vi "LSMcontroller_v61_updatedROIselection.vi"() -> ()   [LabVIEW 2015] (continued)
                  frame False {
                  }
                  frame True {
                    n4769 = local read "Meastab"() -> (w1613:enum32{"X-Y Image", "Linescan", "Timetrace"})
                    n4770 = call "waveformparamsv2.vi"("command"="get") -> ("Params out"=w1619:T15)  [unwired: 4 in, 2 out]
                    n4771 = Unbundle By Name(w1619) -> ("AO parameters"=w1618:T16)
                    n4772 = case shown="\"Timetrace\"" w1613 {
                      tunnel: [w1633 w1634] -> w1612
                      frame "X-Y Image", Default {
                        n4773 = local read "Sampling rate"() -> (w1633:dbl)
                      }
                      frame "Timetrace" {
                        n4774 = local read "srateAODOtt"() -> (w1634:dbl)
                      }
                    }
                    n4775 = Index Array(array=w1618, index=w1616) -> (element=w1617:T17)
                    n4776 = call "waveformsAObuffer.vi"("command"="get") -> ("AO wf out"=w1623:waveform(dbl)[])  [unwired: 1 in]
                    n4777 = call "matlabAOwffromparam.vi"("Cluster"=w1617) -> ("Waveform"=w1621:waveform(dbl))  [unwired: 1 out]
                    n4778 = property on="refwf" class="Ring (strict)"() -> ("RingText.Text"=w1624:string)  [unwired: 2 in, 2 out]
                    n4779 = Replace Array Subset(array=w1623, new element=w1621, index=w1616) -> (w1622:waveform(dbl)[])
                    n4780 = call "waveformsDObuffer.vi"("command"="get") -> ("DO wf out"=w1629:digitalwaveform[])  [unwired: 1 in]
                    n4781 = call "correctwaveformsizetemp.vi"("new sampling frequency (Hz)"=w1612, "start"=FALSE, "reference waveforms to"=w1624, "Analog waveforms in"=w1622, "stop"=FALSE, "Digital waveforms in"=w1629) -> ("analog wf out"=w1627:waveform(dbl)[], "Digital wf out"=w1625:digitalwaveform[], "measpoints"=w1614:i32)
                    n4782 = local read "wavdet"() -> (w1615:bool)
                    n4783 = local write "Analog Lines Plot"(w1627) -> ()
                    n4784 = call "GetNumCamFramesv2.vi"("Digital Waveform Graph"=w1625) -> ("Numeric"=w1626:i32)  [unwired: 10 in]
                    n4785 = local write "Digital Lines Plot"(w1625) -> ()
                    n4786 = call "waveformsAObuffer.vi"("AO wf in"=w1627, "command"="set") -> ()  [unwired: 1 out]
                    n4787 = call "waveformsDObuffer.vi"("DO wf in"=w1625, "command"="set") -> ()  [unwired: 1 out]
                    n4788 = local write "Total Camera Frames"(w1626) -> ()
                    n4789 = case shown="True" w1615 {
                      tunnel: w1614 -> [_ w1635]
                      frame False {
                      }
                      frame True {
                        n4790 = local write "# of frames"(w1635) -> ()
                      }
                    }
                  }
                }
              }
              frame #4 {
                n4791 = local read "finite samples"() -> (w1636:bool)
                n4792 = local read "continuous"() -> (w1637:bool)
                n4793 = local read "wavdet"() -> (w1638:bool)
                n4794 = call "2pparameters.vi"("command"="get") -> ("params out"=w1641:T11)  [unwired: 1 in]
                n4795 = Bundle By Name(cluster=w1641, "finite"=w1636, "cont"=w1637, "wavdet"=w1638) -> (w1639:T11)
                n4796 = call "2pparameters.vi"("Params in"=w1639, "command"="set") -> ()  [unwired: 1 out]
              }
            }
          }
          event "Load Matlab Waveform DO": Value Change {
            n4797 = event-data() -> ()  [unwired: 1 in, 6 out]
            n4798 = stacked-sequence {
              seq-local: [_ _ w1749 _ _] -> [_ _ _ w1764 _]
              seq-local: [_ _ w1748 _ _] -> [_ _ _ w1763 _]
              frame #0 {
                n4799 = local read "Measurement"() -> (w1643:T4)
                n4800 = case shown="\"X-Y-t movie\", Default" w1643 {
                  frame "X-Y-t movie", Default {
                    n4801 = local read "avpp"() -> (w1664:i32)
                    n4802 = local read "Angle ref"() -> (w1663:dbl)
                    n4803 = local read "ROI Type"() -> (w1662:u16)
                    n4804 = local read "xpixels ref"() -> (w1659:i32)
                    n4805 = local read "Vx-min ref"() -> (w1658:dbl)
                    n4806 = local read "Vx-max ref"() -> (w1657:dbl)
                    n4807 = local read "ypixels ref"() -> (w1655:i32)
                    n4808 = local read "Vy-min ref"() -> (w1656:dbl)
                    n4809 = local read "Vy-max ref"() -> (w1652:dbl)
                    n4810 = local read "Sampling rate"() -> (w1646:dbl)
                    n4811 = local read "finite samples"() -> (w1647:bool)
                    n4812 = local read "continuous"() -> (w1650:bool)
                    n4813 = local read "wavdet"() -> (w1651:bool)
                    n4814 = local read "# of frames"() -> (w1649:i32)
                    n4815 = local read "maxbufferAI"() -> (w1648:i32)
                    n4816 = local read "Override AI buffer"() -> (w1644:bool)
                    n4817 = call "2pparameters.vi"("command"="get") -> ("params out"=w1661:T11)  [unwired: 1 in]
                    n4818 = Bundle By Name(cluster=w1661, "type"="X-Y-t movie", "avpp"=w1664, "Angle Img"=w1663, "Xpixels Img"=w1659, "Vx-min Img"=w1658, "VX-max Img"=w1657, "Ypixels Img"=w1655, "Vy-min Img"=w1656, "Vy-max Img"=w1652, "srate"=w1646, "srate Img"=w1646, "finite"=w1647, "cont"=w1650, "wavdet"=w1651, "measpoints"=w1649, "maxbufferAI"=w1648, "Drawing Mode"=w1662, "Vz-reset"=0.0, "AIoverride"=w1644) -> (w1653:T11)
                    n4819 = call "2pparameters.vi"("Params in"=w1653, "command"="set") -> ()  [unwired: 1 out]
                  }
                  frame "X-Y-Z stack" {
                    n4820 = call "2pparameters.vi"("command"="get") -> ("params out"=w1668:T11)  [unwired: 1 in]
                    n4821 = Bundle By Name(cluster=w1668, "type"="X-Y-Z stack") -> (w1666:T11)
                    n4822 = call "2pparameters.vi"("Params in"=w1666, "command"="set") -> ()  [unwired: 1 out]
                  }
                  frame "Lifetime (scan)" {
                    n4823 = call "2pparameters.vi"("command"="get") -> ("params out"=w1673:T11)  [unwired: 1 in]
                    n4824 = Bundle By Name(cluster=w1673, "type"="Lifetime (scan)") -> (w1671:T11)
                    n4825 = call "2pparameters.vi"("Params in"=w1671, "command"="set") -> ()  [unwired: 1 out]
                  }
                  frame "Lifetime (contour)" {
                    n4826 = local read "Vy-min draw"() -> (w1683:dbl)
                    n4827 = local read "Vy-max draw"() -> (w1682:dbl)
                    n4828 = local read "Vx-min draw"() -> (w1685:dbl)
                    n4829 = local read "Vx-max draw"() -> (w1684:dbl)
                    n4830 = local read "xpixels ref"() -> (w1681:i32)
                    n4831 = local read "ypixels ref"() -> (w1680:i32)
                    n4832 = local read "ROI Type"() -> (w1679:u16)
                    n4833 = local read "srateAODOtt"() -> (w1690:dbl)
                    n4834 = local read "# of frames"() -> (w1695:i32)
                    n4835 = local read "refreshtime"() -> (w1687:dbl)
                    n4836 = local read "Pel"() -> (w1678:dbl)
                    n4837 = local read "bin"() -> (w1693:dbl)
                    n4838 = local read "Override AI buffer"() -> (w1676:bool)
                    n4839 = local read "finite samples"() -> (w1702:bool)
                    n4840 = local read "srateAODOtt"() -> (w1689:dbl)
                    n4841 = local read "srateAODOtt"() -> (w1696:dbl)
                    n4842 = local read "continuous"() -> (w1701:bool)
                    n4843 = local read "Angle ref"() -> (w1686:dbl)
                    n4844 = local read "wavdet"() -> (w1703:bool)
                    n4845 = local read "Vx-ref"() -> (w1698:dbl)
                    n4846 = local read "Vy-ref"() -> (w1700:dbl)
                    n4847 = local read "avpp"() -> (w1699:i32)
                    n4848 = call "tt_timeandsamples.vi"("bin"=w1693, "refreshtime"=w1687, "srateAODOtt"=w1690, "tot#ofsamples"=w1695) -> ("refreshrate"=w1691:dbl, "refreshbuffer"=w1692:i32, "timetracecycles"=w1697:i32)  [unwired: 5 in]
                    n4849 = local read "bin"() -> (w1694:dbl)
                    n4850 = call "2pparameters.vi"("command"="get") -> ("params out"=w1706:T11)  [unwired: 1 in]
                    n4851 = Bundle By Name(cluster=w1706, "Drawing Mode"=w1679, "measpoints"=w1695, "tt_cycles"=w1697, "refreshbuffer"=w1692, "refreshrate"=w1691, "Vx-ref"=w1698, "Vy-ref"=w1700, "srate"=w1689, "finite"=w1702, "cont"=w1701, "wavdet"=w1703, "avpp"=w1699, "srateAODO"=w1696, "bufferAI"=w1692, "bin"=w1694, "Angle Img"=w1686, "Vxminref"=w1685, "Vxmaxref"=w1684, "Vyminref"=w1683, "Vymaxref"=w1682, "Xpixels Img"=w1681, "Ypixels Img"=w1680, "Pel"=w1678, "Vz-reset"=0.0, "AIoverride"=w1676, "type"="Lifetime (contour)") -> (w1704:T11)
                    n4852 = Reciprocal(x=w1691) -> (1/x=w1688:dbl)
                    n4853 = local write "refreshtime"(w1688) -> ()
                    n4854 = call "2pparameters.vi"("Params in"=w1704, "command"="set") -> ()  [unwired: 1 out]
                  }
                  frame "X-Y-Z-t movie" {
                  }
                  frame "linescan" {
                  }
                  frame "Timetrace" {
                    n4855 = local read "Vy-min draw"() -> (w1716:dbl)
                    n4856 = local read "Vy-max draw"() -> (w1715:dbl)
                    n4857 = local read "Vx-min draw"() -> (w1718:dbl)
                    n4858 = local read "Vx-max draw"() -> (w1717:dbl)
                    n4859 = local read "xpixels ref"() -> (w1714:i32)
                    n4860 = local read "ypixels ref"() -> (w1713:i32)
                    n4861 = local read "ROI Type"() -> (w1712:u16)
                    n4862 = local read "srateAODOtt"() -> (w1723:dbl)
                    n4863 = local read "# of frames"() -> (w1728:i32)
                    n4864 = local read "refreshtime"() -> (w1720:dbl)
                    n4865 = local read "Pel"() -> (w1711:dbl)
                    n4866 = local read "bin"() -> (w1726:dbl)
                    n4867 = local read "Override AI buffer"() -> (w1709:bool)
                    n4868 = local read "finite samples"() -> (w1735:bool)
                    n4869 = local read "srateAODOtt"() -> (w1722:dbl)
                    n4870 = local read "srateAODOtt"() -> (w1729:dbl)
                    n4871 = local read "continuous"() -> (w1734:bool)
                    n4872 = local read "Angle ref"() -> (w1719:dbl)
                    n4873 = local read "wavdet"() -> (w1736:bool)
                    n4874 = local read "Vx-ref"() -> (w1731:dbl)
                    n4875 = local read "Vy-ref"() -> (w1733:dbl)
                    n4876 = local read "avpp"() -> (w1732:i32)
                    n4877 = call "tt_timeandsamples.vi"("bin"=w1726, "refreshtime"=w1720, "srateAODOtt"=w1723, "tot#ofsamples"=w1728) -> ("refreshrate"=w1724:dbl, "refreshbuffer"=w1725:i32, "timetracecycles"=w1730:i32)  [unwired: 5 in]
                    n4878 = local read "bin"() -> (w1727:dbl)
                    n4879 = call "2pparameters.vi"("command"="get") -> ("params out"=w1739:T11)  [unwired: 1 in]
                    n4880 = Bundle By Name(cluster=w1739, "Drawing Mode"=w1712, "measpoints"=w1728, "tt_cycles"=w1730, "refreshbuffer"=w1725, "refreshrate"=w1724, "Vx-ref"=w1731, "Vy-ref"=w1733, "srate"=w1722, "finite"=w1735, "cont"=w1734, "wavdet"=w1736, "avpp"=w1732, "srateAODO"=w1729, "bufferAI"=w1725, "bin"=w1727, "Angle Img"=w1719, "Vxminref"=w1718, "Vxmaxref"=w1717, "Vyminref"=w1716, "Vymaxref"=w1715, "Xpixels Img"=w1714, "Ypixels Img"=w1713, "Pel"=w1711, "Vz-reset"=0.0, "AIoverride"=w1709, "type"="Timetrace") -> (w1737:T11)
                    n4881 = Reciprocal(x=w1724) -> (1/x=w1721:dbl)
                    n4882 = local write "refreshtime"(w1721) -> ()
                    n4883 = call "2pparameters.vi"("Params in"=w1737, "command"="set") -> ()  [unwired: 1 out]
                  }
                  frame "Lifetime (point)" {
                  }
                }
              }
              frame #1 {
                w1742 = FALSE ("wavdet")
                n4884 = call "2pparameters.vi"("command"="get") -> ("params out"=w1746:T11)  [unwired: 1 in]
                n4885 = Bundle By Name(cluster=w1746, "finite"=w1742, "cont"=w1742, "wavdet"=TRUE) -> (w1743:T11)
                n4886 = call "2pparameters.vi"("Params in"=w1743, "command"="set") -> ()  [unwired: 1 out]
              }
              frame #2 {
                n4887 = local read "DO channels"() -> (w1751:u16)
                n4888 = call "2pparameters.vi"("command"="get") -> ("params out"=w1753:T11)  [unwired: 1 in]
                n4889 = Unbundle By Name(w1753) -> ("aDO"=w1752:u32[])
                n4890 = Search 1D Array(1D array=w1752, element=w1751) -> (index of element=w1749:i32)  [unwired: 1 in]
                n4891 = Greater?(x=w1749, y=-1) -> (0:w1748:bool)
                n4892 = case shown="True" w1748 {
                  tunnel: w1749 -> [_ w1760]
                  frame False {
                  }
                  frame True {
                    n4893 = local read "Meastab"() -> (w1756:enum32{"X-Y Image", "Linescan", "Timetrace"})
                    n4894 = local read "Matlab waveform path DO"() -> (w1758:path)
                    n4895 = local read "Matlab padding value DO"() -> (w1759:dbl)
                    n4896 = case shown="\"Timetrace\"" w1756 {
                      tunnel: [w1761 w1762] -> w1755
                      frame "X-Y Image", Default {
                        n4897 = local read "Sampling rate"() -> (w1761:dbl)
                      }
                      frame "Timetrace" {
                        n4898 = local read "srateAODOtt"() -> (w1762:dbl)
                      }
                    }
                    n4899 = call "matlabwfexistsdialogue.vi"("Matlab waveform path"=w1758) -> ("mtalab waveform path out"=w1757:path)
                    n4900 = call "replace DO matlab param.vi"("Sampling frequency (Hz)"=w1755, "matlab wave number"=w1757, "index of DO wave"=w1760, "padding value"=w1759) -> ()  [unwired: 7 in]
                  }
                }
              }
              frame #3 {
                n4901 = case shown="True" w1763 {
                  tunnel: w1764 -> [_ w1773]
                  frame False {
                  }
                  frame True {
                    n4902 = local read "Meastab"() -> (w1768:enum32{"X-Y Image", "Linescan", "Timetrace"})
                    n4903 = call "waveformparamsv2.vi"("command"="get") -> ("Params out"=w1786:T15)  [unwired: 4 in, 2 out]
                    n4904 = Unbundle By Name(w1786) -> ("DO parameters"=w1785:T18)
                    n4905 = case shown="\"Timetrace\"" w1768 {
                      tunnel: [w1788 w1789] -> w1767
                      frame "X-Y Image", Default {
                        n4906 = local read "Sampling rate"() -> (w1788:dbl)
                      }
                      frame "Timetrace" {
                        n4907 = local read "srateAODOtt"() -> (w1789:dbl)
                      }
                    }
                    n4908 = Index Array(array=w1785, index=w1773) -> (element=w1772:T19)
                    n4909 = call "waveformsDObuffer.vi"("command"="get") -> ("DO wf out"=w1783:digitalwaveform[])  [unwired: 1 in]
                    n4910 = property on="refwf" class="Ring (strict)"() -> ("RingText.Text"=w1775:string)  [unwired: 2 in, 2 out]
                    n4911 = call "matlabDOwffromparam.vi"("waveform params"=w1772) -> ("digital waveform"=w1771:digitalwaveform)
                    n4912 = Replace Array Subset(array=w1783, new element=w1771, index=w1773) -> (w1774:digitalwaveform[])
                    n4913 = call "waveformsAObuffer.vi"("command"="get") -> ("AO wf out"=w1782:waveform(dbl)[])  [unwired: 1 in]
                    n4914 = local read "wavdet"() -> (w1770:bool)
                    n4915 = call "correctwaveformsizetemp.vi"("new sampling frequency (Hz)"=w1767, "start"=FALSE, "reference waveforms to"=w1775, "Analog waveforms in"=w1782, "stop"=FALSE, "Digital waveforms in"=w1774) -> ("analog wf out"=w1778:waveform(dbl)[], "Digital wf out"=w1776:digitalwaveform[], "measpoints"=w1769:i32)
                    n4916 = local write "Analog Lines Plot"(w1778) -> ()
                    n4917 = call "GetNumCamFramesv2.vi"("Digital Waveform Graph"=w1776) -> ("Numeric"=w1777:i32)  [unwired: 10 in]
                    n4918 = local write "Digital Lines Plot"(w1776) -> ()
                    n4919 = case shown="True" w1770 {
                      tunnel: w1769 -> [_ w1790]
                      frame False {
                      }
                      frame True {
                        n4920 = local write "# of frames"(w1790) -> ()
                      }
                    }
                    n4921 = call "waveformsAObuffer.vi"("AO wf in"=w1778, "command"="set") -> ()  [unwired: 1 out]
                    n4922 = call "waveformsDObuffer.vi"("DO wf in"=w1776, "command"="set") -> ()  [unwired: 1 out]
                    n4923 = local write "Total Camera Frames"(w1777) -> ()
                  }
                }
              }
              frame #4 {
                n4924 = local read "finite samples"() -> (w1791:bool)
                n4925 = local read "continuous"() -> (w1792:bool)
                n4926 = local read "wavdet"() -> (w1793:bool)
                n4927 = call "2pparameters.vi"("command"="get") -> ("params out"=w1796:T11)  [unwired: 1 in]
                n4928 = Bundle By Name(cluster=w1796, "finite"=w1791, "cont"=w1792, "wavdet"=w1793) -> (w1794:T11)
                n4929 = call "2pparameters.vi"("Params in"=w1794, "command"="set") -> ()  [unwired: 1 out]
              }
            }
          }
          event "Add settings": Value Change {
            n4930 = event-data() -> ()  [unwired: 1 in, 6 out]
            n4931 = call "wfsettings.vi"("command"="get") -> ("wfsettings out"=w1800:T29)  [unwired: 2 in, 1 out]
            n4932 = in-place {
              n4933 = in-place-cluster #53(w1800) -> ("settings names"=w1805:string[], "settings locations"=w1807:path[])
              n4934 = local read "Setting location"() -> (w1803:path)
              n4935 = local read "Nickname"() -> (w1802:string)
              n4936 = Build Array (concatenate)(w1805, w1802) -> (w1804:string[])
              n4937 = property on="Loaded settings" class="Ring (strict)"("Strings []"=w1804) -> ()  [unwired: 2 in, 2 out]
              n4938 = Build Array (concatenate)(w1807, w1803) -> (w1806:path[])
              n4939 = in-place-cluster #53("settings names"=w1804, "settings locations"=w1806) -> (w1798:T29)
            }
            n4940 = call "wfsettings.vi"("wfsettings in"=w1798, "command"="set") -> ()  [unwired: 1 in, 2 out]
          }
          event "Rem setting": Value Change {
            n4941 = event-data() -> ()  [unwired: 1 in, 6 out]
            n4942 = call "wfsettings.vi"("command"="get") -> ("wfsettings out"=w1810:T29)  [unwired: 2 in, 1 out]
            n4943 = in-place {
              n4944 = in-place-cluster #54(w1810) -> ("settings names"=w1815:string[], "settings locations"=w1813:path[])
              n4945 = property on="Loaded settings" class="Ring (strict)"() -> ("RingText.Text"=w1816:string)  [unwired: 2 in, 2 out]
              n4946 = Search 1D Array(1D array=w1815, element=w1816) -> (index of element=w1817:i32)  [unwired: 1 in]
              n4947 = Delete From Array(array=w1815, index=w1817) -> (array with subset deleted=w1814:string[])  [unwired: 1 in, 1 out]
              n4948 = Delete From Array(array=w1813, index=w1817) -> (array with subset deleted=w1812:path[])  [unwired: 1 in, 1 out]
              n4949 = property on="Loaded settings" class="Ring (strict)"("Strings []"=w1814) -> ()  [unwired: 2 in, 2 out]
              n4950 = in-place-cluster #54("settings names"=w1814, "settings locations"=w1812) -> (w1808:T29)
            }
            n4951 = call "wfsettings.vi"("wfsettings in"=w1808, "command"="set") -> ()  [unwired: 1 in, 2 out]
          }
          event "Update settings": Value Change {
            n4952 = event-data() -> ()  [unwired: 1 in, 6 out]
            n4953 = stacked-sequence {
              frame #0 {
                n4954 = local read "Measurement"() -> (w1818:T4)
                n4955 = case shown="\"Timetrace\"" w1818 {
                  frame "X-Y-t movie", Default {
                    n4956 = local read "avpp"() -> (w1839:i32)
                    n4957 = local read "Angle ref"() -> (w1838:dbl)
                    n4958 = local read "ROI Type"() -> (w1837:u16)
                    n4959 = local read "xpixels ref"() -> (w1834:i32)
                    n4960 = local read "Vx-min ref"() -> (w1833:dbl)
                    n4961 = local read "Vx-max ref"() -> (w1832:dbl)
                    n4962 = local read "ypixels ref"() -> (w1830:i32)
                    n4963 = local read "Vy-min ref"() -> (w1831:dbl)
                    n4964 = local read "Vy-max ref"() -> (w1827:dbl)
                    n4965 = local read "Sampling rate"() -> (w1821:dbl)
                    n4966 = local read "finite samples"() -> (w1822:bool)
                    n4967 = local read "continuous"() -> (w1825:bool)
                    n4968 = local read "wavdet"() -> (w1826:bool)
                    n4969 = local read "# of frames"() -> (w1824:i32)
                    n4970 = local read "maxbufferAI"() -> (w1823:i32)
                    n4971 = local read "Override AI buffer"() -> (w1819:bool)
                    n4972 = call "2pparameters.vi"("command"="get") -> ("params out"=w1836:T11)  [unwired: 1 in]
                    n4973 = Bundle By Name(cluster=w1836, "type"="X-Y-t movie", "avpp"=w1839, "Angle Img"=w1838, "Xpixels Img"=w1834, "Vx-min Img"=w1833, "VX-max Img"=w1832, "Ypixels Img"=w1830, "Vy-min Img"=w1831, "Vy-max Img"=w1827, "srate"=w1821, "srate Img"=w1821, "finite"=w1822, "cont"=w1825, "wavdet"=w1826, "measpoints"=w1824, "maxbufferAI"=w1823, "Drawing Mode"=w1837, "Vz-reset"=0.0, "AIoverride"=w1819) -> (w1828:T11)
                    n4974 = call "2pparameters.vi"("Params in"=w1828, "command"="set") -> ()  [unwired: 1 out]
                  }
                  frame "X-Y-Z stack" {
                    n4975 = call "2pparameters.vi"("command"="get") -> ("params out"=w1843:T11)  [unwired: 1 in]
                    n4976 = Bundle By Name(cluster=w1843, "type"="X-Y-Z stack") -> (w1841:T11)
                    n4977 = call "2pparameters.vi"("Params in"=w1841, "command"="set") -> ()  [unwired: 1 out]
                  }
                  frame "Lifetime (scan)" {
                    n4978 = call "2pparameters.vi"("command"="get") -> ("params out"=w1848:T11)  [unwired: 1 in]
                    n4979 = Bundle By Name(cluster=w1848, "type"="Lifetime (scan)") -> (w1846:T11)
                    n4980 = call "2pparameters.vi"("Params in"=w1846, "command"="set") -> ()  [unwired: 1 out]
                  }
                  frame "Lifetime (contour)" {
                    n4981 = local read "Vy-min draw"() -> (w1858:dbl)
                    n4982 = local read "Vy-max draw"() -> (w1857:dbl)
                    n4983 = local read "Vx-min draw"() -> (w1860:dbl)
                    n4984 = local read "Vx-max draw"() -> (w1859:dbl)
                    n4985 = local read "xpixels ref"() -> (w1856:i32)
                    n4986 = local read "ypixels ref"() -> (w1855:i32)
                    n4987 = local read "ROI Type"() -> (w1854:u16)
                    n4988 = local read "srateAODOtt"() -> (w1865:dbl)
                    n4989 = local read "# of frames"() -> (w1870:i32)
                    n4990 = local read "refreshtime"() -> (w1862:dbl)
                    n4991 = local read "Pel"() -> (w1853:dbl)
                    n4992 = local read "bin"() -> (w1868:dbl)
                    n4993 = local read "Override AI buffer"() -> (w1851:bool)
                    n4994 = local read "finite samples"() -> (w1877:bool)
                    n4995 = local read "srateAODOtt"() -> (w1864:dbl)
                    n4996 = local read "srateAODOtt"() -> (w1871:dbl)
                    n4997 = local read "continuous"() -> (w1876:bool)
                    n4998 = local read "Angle ref"() -> (w1861:dbl)
                    n4999 = local read "wavdet"() -> (w1878:bool)
                    n5000 = local read "Vx-ref"() -> (w1873:dbl)
                    n5001 = local read "Vy-ref"() -> (w1875:dbl)
                    n5002 = local read "avpp"() -> (w1874:i32)
                    n5003 = call "tt_timeandsamples.vi"("bin"=w1868, "refreshtime"=w1862, "srateAODOtt"=w1865, "tot#ofsamples"=w1870) -> ("refreshrate"=w1866:dbl, "refreshbuffer"=w1867:i32, "timetracecycles"=w1872:i32)  [unwired: 5 in]
                    n5004 = local read "bin"() -> (w1869:dbl)
                    n5005 = call "2pparameters.vi"("command"="get") -> ("params out"=w1881:T11)  [unwired: 1 in]
                    n5006 = Bundle By Name(cluster=w1881, "Drawing Mode"=w1854, "measpoints"=w1870, "tt_cycles"=w1872, "refreshbuffer"=w1867, "refreshrate"=w1866, "Vx-ref"=w1873, "Vy-ref"=w1875, "srate"=w1864, "finite"=w1877, "cont"=w1876, "wavdet"=w1878, "avpp"=w1874, "srateAODO"=w1871, "bufferAI"=w1867, "bin"=w1869, "Angle Img"=w1861, "Vxminref"=w1860, "Vxmaxref"=w1859, "Vyminref"=w1858, "Vymaxref"=w1857, "Xpixels Img"=w1856, "Ypixels Img"=w1855, "Pel"=w1853, "Vz-reset"=0.0, "AIoverride"=w1851, "type"="Lifetime (contour)") -> (w1879:T11)
                    n5007 = Reciprocal(x=w1866) -> (1/x=w1863:dbl)
                    n5008 = local write "refreshtime"(w1863) -> ()
                    n5009 = call "2pparameters.vi"("Params in"=w1879, "command"="set") -> ()  [unwired: 1 out]
                  }
                  frame "X-Y-Z-t movie" {
                  }
                  frame "linescan" {
                  }
                  frame "Timetrace" {
                    n5010 = local read "Vy-min draw"() -> (w1891:dbl)
                    n5011 = local read "Vy-max draw"() -> (w1890:dbl)
                    n5012 = local read "Vx-min draw"() -> (w1893:dbl)
                    n5013 = local read "Vx-max draw"() -> (w1892:dbl)
                    n5014 = local read "xpixels ref"() -> (w1889:i32)
                    n5015 = local read "ypixels ref"() -> (w1888:i32)
                    n5016 = local read "ROI Type"() -> (w1887:u16)
                    n5017 = local read "srateAODOtt"() -> (w1898:dbl)
                    n5018 = local read "# of frames"() -> (w1903:i32)
                    n5019 = local read "refreshtime"() -> (w1895:dbl)
                    n5020 = local read "Pel"() -> (w1886:dbl)
                    n5021 = local read "bin"() -> (w1901:dbl)
                    n5022 = local read "Override AI buffer"() -> (w1884:bool)
                    n5023 = local read "finite samples"() -> (w1910:bool)
                    n5024 = local read "srateAODOtt"() -> (w1897:dbl)
                    n5025 = local read "srateAODOtt"() -> (w1904:dbl)
                    n5026 = local read "continuous"() -> (w1909:bool)
                    n5027 = local read "Angle ref"() -> (w1894:dbl)
                    n5028 = local read "wavdet"() -> (w1911:bool)
                    n5029 = local read "Vx-ref"() -> (w1906:dbl)
                    n5030 = local read "Vy-ref"() -> (w1908:dbl)
                    n5031 = local read "avpp"() -> (w1907:i32)
                    n5032 = call "tt_timeandsamples.vi"("bin"=w1901, "refreshtime"=w1895, "srateAODOtt"=w1898, "tot#ofsamples"=w1903) -> ("refreshrate"=w1899:dbl, "refreshbuffer"=w1900:i32, "timetracecycles"=w1905:i32)  [unwired: 5 in]
                    n5033 = local read "bin"() -> (w1902:dbl)
                    n5034 = call "2pparameters.vi"("command"="get") -> ("params out"=w1914:T11)  [unwired: 1 in]
                    n5035 = Bundle By Name(cluster=w1914, "Drawing Mode"=w1887, "measpoints"=w1903, "tt_cycles"=w1905, "refreshbuffer"=w1900, "refreshrate"=w1899, "Vx-ref"=w1906, "Vy-ref"=w1908, "srate"=w1897, "finite"=w1910, "cont"=w1909, "wavdet"=w1911, "avpp"=w1907, "srateAODO"=w1904, "bufferAI"=w1900, "bin"=w1902, "Angle Img"=w1894, "Vxminref"=w1893, "Vxmaxref"=w1892, "Vyminref"=w1891, "Vymaxref"=w1890, "Xpixels Img"=w1889, "Ypixels Img"=w1888, "Pel"=w1886, "Vz-reset"=0.0, "AIoverride"=w1884, "type"="Timetrace") -> (w1912:T11)
                    n5036 = Reciprocal(x=w1899) -> (1/x=w1896:dbl)
                    n5037 = local write "refreshtime"(w1896) -> ()
                    n5038 = call "2pparameters.vi"("Params in"=w1912, "command"="set") -> ()  [unwired: 1 out]
                  }
                  frame "Lifetime (point)" {
                  }
                }
              }
              frame #1 {
                w1917 = FALSE ("wavdet")
                n5039 = call "2pparameters.vi"("command"="get") -> ("params out"=w1921:T11)  [unwired: 1 in]
                n5040 = Bundle By Name(cluster=w1921, "finite"=w1917, "cont"=w1917, "wavdet"=TRUE) -> (w1918:T11)
                n5041 = call "2pparameters.vi"("Params in"=w1918, "command"="set") -> ()  [unwired: 1 out]
              }
              frame #2 {
                n5042 = property on="Loaded settings" class="Ring (strict)"() -> ("RingText.Text"=w1923:string)  [unwired: 2 in, 2 out]
                n5043 = control-ref of="Analog Lines Plot"() -> (w1925:refnum<vi>)
                n5044 = control-ref of="Digital Lines Plot"() -> (w1924:refnum<vi>)
                n5045 = call "Usedlinesfromsettingsfile.vi"("sertting"=w1923) -> ("used AO names"=w1929:string[], "used AO lines"=w1928:tag[], "used DO names"=w1927:string[], "used DO lines"=w1926:tag[])
                n5046 = call "loadAODOwfparamsfromsettingsfile.vi"("sertting"=w1923) -> ()
                n5047 = call "prepAOWaveplot.vi"("WaveformGraph in"=w1925, "Analog Used Names"=w1929) -> ()  [unwired: 1 in]
                n5048 = local write "Analog Used Names"(w1929) -> ()
                n5049 = local write "Analog Used Lines"(w1928) -> ()
                n5050 = call "prepDOWaveplot.vi"("DigitalGraph in"=w1924, "used DO names"=w1927) -> ()  [unwired: 1 in]
                n5051 = local write "Digital Used Names"(w1927) -> ()
                n5052 = local write "Digital Used Lines"(w1926) -> ()
              }
              frame #3 {
                n5053 = call "waveformparamsv2.vi"("command"="get") -> ("Params out"=w1946:T15)  [unwired: 4 in, 2 out]
                n5054 = Unbundle By Name(w1946) -> ("AO parameters"=w1947:T16, "DO parameters"=w1948:T18)
                n5055 = for {
                  tunnel: w1947 -> [w1967] mode=indexing
                  tunnel: [w1965] -> w1949 mode=indexing
                  tunnel: [w1964] -> w1934 mode=indexing
                  tunnel: [w1962] -> w1937 mode=indexing
                  i -> [w1966]
                  n5056 = Unbundle By Name(w1967) -> ("AOtab"=w1968:dbl)
                  n5057 = case shown="0, Default" w1968 {
                    tunnel: w1967 -> [_ w1979 w1981 w1983]
                    tunnel: [_ w1978 w1980 w1982] -> w1963
                    frame -1 {
                    }
                    frame 0, Default {
                      n5058 = call "generateRampedSquareWave_fromAOparameters.vi"("AO params"=w1979) -> ("Waveform"=w1978:waveform(dbl))  [unwired: 1 out]
                    }
                    frame 1 {
                      n5059 = call "generateTriWave_fromAOparameters.vi"("AO params"=w1981) -> ("Waveform"=w1980:waveform(dbl))  [unwired: 1 out]
                    }
                    frame 2 {
                      n5060 = call "matlabAOwffromparam.vi"("Cluster"=w1983) -> ("Waveform"=w1982:waveform(dbl))  [unwired: 1 out]
                    }
                  }
                  n5061 = case shown="0" w1966 {
                    tunnel: [w1973 -1] -> w1965
                    tunnel: [w1972 w1976] -> w1964
                    tunnel: w1963 -> [w1972 w1976]
                    tunnel: [w1969 -1.0] -> w1962
                    frame 0 {
                      n5062 = Unbundle By Name(w1972) -> ("dt"=w1971:dbl, "Y"=w1974:dbl[])
                      n5063 = Reciprocal(x=w1971) -> (1/x=w1970:dbl)
                      n5064 = Array Size(array=w1974) -> (size(s)=w1973:i32)
                      n5065 = Round To Nearest(number=w1970) -> (nearest integer value=w1969:dbl)
                    }
                    frame 1, Default {
                    }
                  }
                }
                n5066 = Index Array(array=w1949, index=0) -> (element=w1951:i32)
                n5067 = Index Array(array=w1937, index=0) -> (element=w1936:dbl)
                n5068 = for {
                  tunnel: w1948 -> [w1956] mode=indexing
                  tunnel: [w1954] -> w1935 mode=indexing
                  tunnel: w1951 -> [w1953]
                  n5069 = Unbundle By Name(w1956) -> ("DOtab"=w1955:dbl)
                  n5070 = case shown="0, Default" w1955 {
                    tunnel: w1956 -> [w1959 w1961]
                    tunnel: w1953 -> [w1958 _]
                    tunnel: [w1957 w1960] -> w1954
                    frame 0, Default {
                      n5071 = call "simple digital from wf params.vi"("waveform params"=w1959, "number of samples"=w1958) -> ("digital waveform"=w1957:digitalwaveform)
                    }
                    frame 1 {
                      n5072 = call "matlabDOwffromparam.vi"("waveform params"=w1961) -> ("digital waveform"=w1960:digitalwaveform)
                    }
                  }
                }
                n5073 = property on="refwf" class="Ring (strict)"() -> ("RingText.Text"=w1939:string)  [unwired: 2 in, 2 out]
                n5074 = call "correctwaveformsizetemp.vi"("new sampling frequency (Hz)"=w1936, "start"=FALSE, "reference waveforms to"=w1939, "Analog waveforms in"=w1934, "stop"=FALSE, "Digital waveforms in"=w1935) -> ("analog wf out"=w1933:waveform(dbl)[], "Digital wf out"=w1932:digitalwaveform[], "measpoints"=w1930:i32)
                n5075 = local read "wavdet"() -> (w1931:bool)
                n5076 = case shown="True" w1931 {
                  tunnel: w1930 -> [_ w1952]
                  frame False {
                  }
                  frame True {
                    n5077 = local write "# of frames"(w1952) -> ()
                  }
                }
                n5078 = local write "Analog Lines Plot"(w1933) -> ()
                n5079 = local write "Digital Lines Plot"(w1932) -> ()
                n5080 = call "GetNumCamFramesv2.vi"("Digital Waveform Graph"=w1932) -> ("Numeric"=w1944:i32)  [unwired: 10 in]
                n5081 = call "waveformsAObuffer.vi"("AO wf in"=w1933, "command"="set") -> ()  [unwired: 1 out]
                n5082 = call "waveformsDObuffer.vi"("DO wf in"=w1932, "command"="set") -> ()  [unwired: 1 out]
                n5083 = local write "Total Camera Frames"(w1944) -> ()
              }
              frame #4 {
                n5084 = local read "AO channels"() -> (w1984:u32)
                n5085 = call "2pparameters.vi"("command"="get") -> ("params out"=w1986:T11)  [unwired: 1 in]
                n5086 = Unbundle By Name(w1986) -> ("aAO"=w1985:u32[])
                n5087 = Search 1D Array(1D array=w1985, element=w1984) -> (index of element=w1988:i32)  [unwired: 1 in]
                n5088 = Equal?(x=w1988, y=-1.0) -> (x = y?=w1989:bool)
                n5089 = case shown="False" w1989 {
                  tunnel: w1988 -> [w2014 _]
                  frame False {
                    n5090 = call "waveformparamsv2.vi"("command"="get") -> ("Params out"=w1997:T15)  [unwired: 4 in, 2 out]
                    n5091 = Unbundle By Name(w1997) -> ("AO parameters"=w1996:T16)
                    n5092 = Index Array(array=w1996, index=w2014) -> (element=w2013:T17)
                    n5093 = Unbundle By Name(w2013) -> ("AOtab"=w1994:dbl, "Repeats"=w2012:dbl, "Cycles"=w2011:dbl, "Start amplitude (V)"=w2010:dbl, "Baseline (V)"=w2009:dbl, "Step size (V)"=w2008:dbl, "DC (%)"=w2007:dbl, "Sampling frequency (Hz)"=w2006:dbl, "Period (ms)"=w2005:dbl, "Offset (V)"=w2004:dbl, "Amplitude (V)"=w2003:dbl, "Frequency"=w2002:dbl, "Tri Repeats"=w2001:dbl, "phase shift (ms)"=w2000:dbl, "Pulses"=w1999:dbl, "Tri phase"=w1995:dbl, "padding value"=w1991:dbl, "Matlab wave file"=w1992:path)
                    n5094 = To Unsigned Long Integer(number=w1994) -> (unsigned 32bit integer=w1993:u32)
                    n5095 = local write "Build analog waveform tabs"(w1993) -> ()
                    n5096 = local write "Matlab waveform path"(w1992) -> ()
                    n5097 = local write "phase shift (ms)"(w2000) -> ()
                    n5098 = local write "Repeats"(w2012) -> ()
                    n5099 = local write "Cycles"(w2011) -> ()
                    n5100 = local write "Amplitude (V)"(w2003) -> ()
                    n5101 = local write "Matlab padding value"(w1991) -> ()
                    n5102 = local write "Tri padding value"(w1991) -> ()
                    n5103 = local write "Start amplitude (V)"(w2010) -> ()
                    n5104 = local write "Tri Phase (s)"(w1995) -> ()
                    n5105 = local write "Period (ms)"(w2005) -> ()
                    n5106 = local write "Tri Repeats"(w2001) -> ()
                    n5107 = local write "Offset (V)"(w2004) -> ()
                    n5108 = local write "Frequency"(w2002) -> ()
                    n5109 = local write "Pulses"(w1999) -> ()
                    n5110 = local write "padding value"(w1991) -> ()
                    n5111 = local write "Sampling rate \ncurrent wf"(w2006) -> ()
                    n5112 = local write "Baseline (V)"(w2009) -> ()
                    n5113 = local write "Step size (V)"(w2008) -> ()
                    n5114 = local write "DC (%)"(w2007) -> ()
                  }
                  frame True {
                  }
                }
              }
              frame #5 {
                n5115 = local read "DO channels"() -> (w2017:u16)
                n5116 = call "2pparameters.vi"("command"="get") -> ("params out"=w2019:T11)  [unwired: 1 in]
                n5117 = Unbundle By Name(w2019) -> ("aDO"=w2018:u32[])
                n5118 = Search 1D Array(1D array=w2018, element=w2017) -> (index of element=w2016:i32)  [unwired: 1 in]
                n5119 = Equal?(x=w2016, y=-1.0) -> (x = y?=w2015:bool)
                n5120 = case shown="False" w2015 {
                  tunnel: w2016 -> [w2034 _]
                  frame False {
                    n5121 = call "waveformparamsv2.vi"("command"="get") -> ("Params out"=w2028:T15)  [unwired: 4 in, 2 out]
                    n5122 = Unbundle By Name(w2028) -> ("DO parameters"=w2026:T18)
                    n5123 = Index Array(array=w2026, index=w2034) -> (element=w2033:T19)
                    n5124 = Unbundle By Name(w2033) -> ("Digital DC (%)"=w2032:dbl, "Digital phase"=w2031:dbl, "Digital Freq (Hz)"=w2030:dbl, "Sampling frequency (Hz)"=w2029:dbl, "Digital time offset (s)"=w2025:dbl, "padding value"=w2024:dbl, "matlab wave file"=w2023:path, "DOtab"=w2022:dbl)
                    n5125 = local write "Build digital waveform tabs"(w2022) -> ()
                    n5126 = local write "Digital DC (%)"(w2032) -> ()
                    n5127 = local write "Matlab waveform path DO"(w2023) -> ()
                    n5128 = local write "Sampling rate \ncurrent wf"(w2029) -> ()
                    n5129 = local write "Digital time offset (s)"(w2025) -> ()
                    n5130 = local write "Matlab padding value DO"(w2024) -> ()
                    n5131 = local write "Digital padding value"(w2024) -> ()
                    n5132 = local write "Digital Freq (Hz)"(w2030) -> ()
                    n5133 = local write "Digital phase (s)"(w2031) -> ()
                  }
                  frame True {
                  }
                }
              }
              frame #6 {
                n5134 = local read "finite samples"() -> (w2035:bool)
                n5135 = local read "continuous"() -> (w2036:bool)
                n5136 = local read "wavdet"() -> (w2037:bool)
                n5137 = call "2pparameters.vi"("command"="get") -> ("params out"=w2040:T11)  [unwired: 1 in]
                n5138 = Bundle By Name(cluster=w2040, "finite"=w2035, "cont"=w2036, "wavdet"=w2037) -> (w2038:T11)
                n5139 = call "2pparameters.vi"("Params in"=w2038, "command"="set") -> ()  [unwired: 1 out]
              }
            }
          }
          event "Exit": Value Change {
            n5140 = event-data() -> ("NewVal"=w2042:bool)  [unwired: 1 in]
          }
        }
        n5141 = Wait (ms)(milliseconds to wait=u32 50) -> ()  [unwired: 1 out]
      }
    }
    frame #3 {
      w6617 = FALSE ("Value (Signaling)")
      n5142 = property on="Start" class="Bool (strict)"("Val(Sgnl)"=w6617) -> ()  [unwired: 2 in, 2 out]
      n5143 = property on="Exit" class="Bool (strict)"("Val(Sgnl)"=w6617) -> ()  [unwired: 2 in, 2 out]
      n5144 = property on="Stop" class="Bool (strict)"("Val(Sgnl)"=w6617) -> ()  [unwired: 2 in, 2 out]
      n5145 = flat-sequence {
        frame #0 {
          w6618 = u16 1 items=["OD 0"=1, "OD 0.5"=2, "OD 1"=3, "OD 2"=4, "OD 3"=5, "OD 4"=6] ("New ODfilt")
          n5146 = local read "ODfilt"() -> (w6619:u16)
          n5147 = call "filterwheelcontrol_nothorlabslib.vi"("Current OD filt"=w6619, "New ODfilt"=w6618) -> ()  [unwired: 1 in]
        }
        frame #1 {
          n5148 = Wait (ms)(milliseconds to wait=u32 1000) -> ()  [unwired: 1 out]
        }
      }
    }
  }
